vi "PicoScope4000ExampleBlock.vi"() -> ()   [LabVIEW 2010]
panel:
  in  "Acquisition Settings":T1={"preTriggerSamples"=0, "postTriggerSamples"=1000, "timebase"=2, "Aggregate Data"=FALSE, "Down Sample Ratio"=1, "Four Channel Device"=FALSE, "Oversample"=1} {"Down Sample Ratio" min=1 step=1}
  in  "Trigger Settings":T2={"Trigger Enabled"=FALSE, "Trigger Source"=enum."Channel A", "Trigger Threshold (16-bit counts)"=0, "Trigger Direction"=2, "Trigger Delay (samples)"=0, "Auto Trigger Time (ms)"=1000} {"Trigger Direction" items=["Rising"=2, "Falling"=3]}
  in  "Channel A Settings":T3={"Enabled"=TRUE, "DC Coupled"=TRUE, "Range"=6} {"Range" items=["10 mV", "20 mV", "50 mV", "100 mV", "200 mV", "500 mV", "1 V", "2 V", "5 V", "10 V", "20 V", "50 V ", "100 V"]}
  in  "stop":bool
  out "Channel A":i16[](graph)
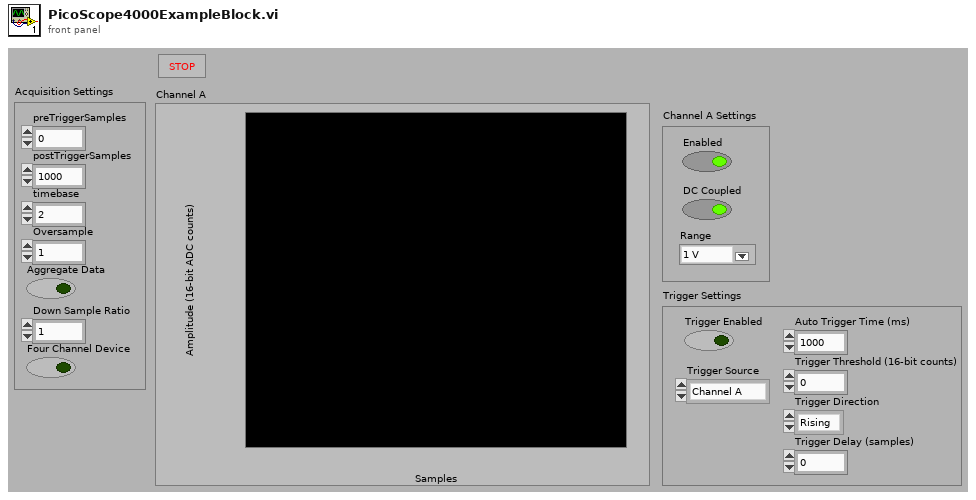
[diagram p1: front panel]
types:
  T1 = cluster{"preTriggerSamples":i32, "postTriggerSamples":i32, "timebase":u32, "Aggregate Data":bool, "Down Sample Ratio":u32, "Four Channel Device":bool, "Oversample":i16}
  T2 = cluster{"Trigger Enabled":bool, "Trigger Source":enum16{"Channel A", "Channel B", "Channel C", "Channel D", "Ext"}, "Trigger Threshold (16-bit counts)":i16, "Trigger Direction":u16, "Trigger Delay (samples)":u32, "Auto Trigger Time (ms)":i16}
  T3 = cluster{"Enabled":bool, "DC Coupled":bool, "Range":u16}
  T4 = cluster{"Channel D Buffer":i16[], "Channel C Buffer":i16[], "Channel B Buffer":i16[], "Channel A Buffer":i16[]}
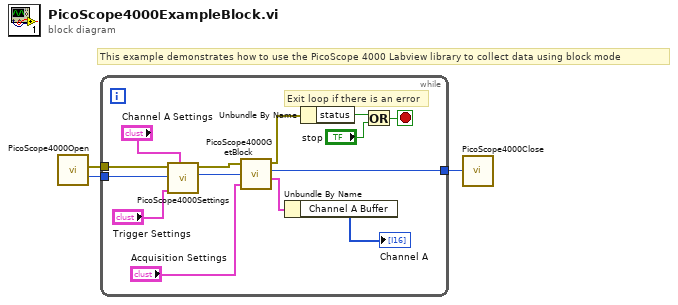
[diagram p0: block diagram]
diagram:
  # "This example demonstrates how to use the PicoScope 4000 Labview library to collect data using block mode"
  n1 = call "PicoScope4000Open.vi"() -> ("error out"=w3:errorcluster, "handle"=w2:i16)  [unwired: 1 in]
  n2 = while {
    tunnel: w2 -> [w17]
    tunnel: [w7] -> w1
    tunnel: w3 -> [w16]
    stop <- w14 stop-if-true
    # "Exit loop if there is an error"
    n3 = call "PicoScope4000Settings.vi"("Channel A Settings"="Channel A Settings", "Trigger Settings"="Trigger Settings", "handle in"=w17, "error in"=w16) -> ("handle out"=w9:i16, "error out"=w8:errorcluster)  [unwired: 6 in]
    n4 = call "PicoScope4000GetBlock.vi"("error in"=w8, "handle in"=w9, "Acquisition Settings"="Acquisition Settings") -> ("error out"=w6:errorcluster, "handle out"=w7:i16, "Buffers (Max or non-aggregated)"=w5:T4)  [unwired: 3 in, 2 out]
    n5 = Unbundle By Name(w5) -> ("Channel A Buffer"=→"Channel A":i16[])
    n6 = Unbundle By Name(w6) -> ("status"=w13:bool)
    n7 = Or(x=w13, y="stop") -> (x .or. y?=w14:bool)
  }
  n8 = call "PicoScope4000Close.vi"("handle"=w1) -> ()
